vi "Read Prep No Objects.vi"(8 "error in (no error)":errorcluster, 11 "Photon Counter SR 400 in":T1={"Mode"=0, "Count Time"=0.0, "Trigger Frequency"=10000000.0, "Trigger External?"=FALSE, "Gate A Mode"=0, "Gate A Width"=0.0, "Gate A Delay"=0.0, "Gate B Mode"=0, "Gate B Width"=0.0, "Gate B Delay"=0.0} {"Mode" items=["A,B For T Preset", "A-B For T Preset", "A+B For T Preset", "A For B Preset"]; "Gate A Mode" items=["CW", "Fixed"]; "Gate B Mode" items=["CW", "Fixed"]}) -> (0 "error out":errorcluster, 3 "Photon Counter SR 400 out":T1={"Mode"=0, "Count Time"=0.0, "Trigger Frequency"=10000000.0, "Trigger External?"=FALSE, "Gate A Mode"=0, "Gate A Width"=0.0, "Gate A Delay"=0.0, "Gate B Mode"=0, "Gate B Width"=0.0, "Gate B Delay"=0.0} {"Mode" items=["A,B For T Preset", "A-B For T Preset", "A+B For T Preset", "A For B Preset"]; "Gate A Mode" items=["CW", "Fixed"]; "Gate B Mode" items=["CW", "Fixed"]})   [LabVIEW 2012]
doc: "This is in case the readable object needs to change some settings before the time delay occurs. One example: if the photon counter needs to change the gates, e.g. to track the current pulse settings."
uses:
  Global/GPIB Numbers.vi
  SR400/SR400.lvlib
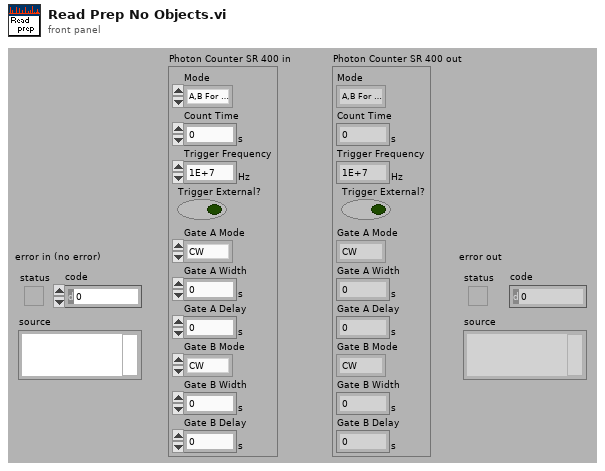
[diagram p1: front panel]
types:
  T1 = cluster{"Mode":u16, "Count Time":dbl[unit], "Trigger Frequency":dbl[unit], "Trigger External?":bool, "Gate A Mode":u16, "Gate A Width":dbl[unit], "Gate A Delay":dbl[unit], "Gate B Mode":u16, "Gate B Width":dbl[unit], "Gate B Delay":dbl[unit]}
  T2 = typedef "GPIB Type Def.ctl" = cluster{"Name":string, "bus":dbl, "GPIB":dbl, "GPIB as string":string, "byte":i32, "VISA Resource Name":refnum<visa-resource-name>}
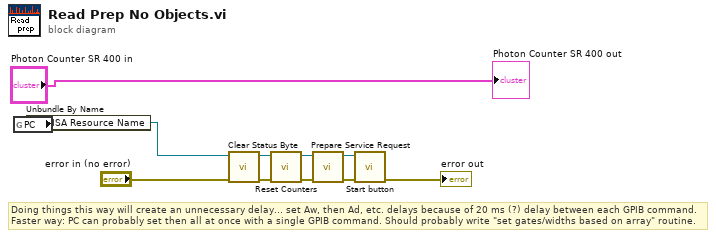
[diagram p0: block diagram]
diagram:
  # "Doing things this way will create an unnecessary delay... set Aw, then Ad, etc. delays because of 20 ms (?) delay between each GPIB command.\nFaster way: PC can probably set then all at once with a single GPIB command. Should probably write \"set gates/widths based on array\" routine."
  n1 = global read "GPIB Numbers.vi" "PC"() -> (w2:T2)
  n2 = Unbundle By Name(w2) -> ("VISA Resource Name"=w1:refnum<visa-resource-name>)
  n3 = call "Clear Status Byte.vi"("error in (no error)"="error in (no error)", "VISA resource name"=w1) -> ("error out"=w8:errorcluster, "VISA resource name out"=w11:refnum<visa-resource-name>)  [unwired: 8 out]
  n4 = call "Reset Counters.vi"("error in (no error)"=w8, "VISA resource name"=w11) -> ("error out"=w7:errorcluster, "VISA resource name out"=w10:refnum<visa-resource-name>)  [unwired: 8 out]
  n5 = call "Prepare Service Request.vi"("error in (no error)"=w7, "VISA resource name"=w10) -> ("error out"=w6:errorcluster, "VISA resource name out"=w9:refnum<visa-resource-name>)  [unwired: 1 in, 7 out]
  n6 = call "Start button.vi"("error in (no error)"=w6, "VISA resource name"=w9) -> ("error out"=→"error out":errorcluster)  [unwired: 9 out]
  "Photon Counter SR 400 out" <- "Photon Counter SR 400 in"
